vi "DemoApplication_Create.vi"(8 "Error In":errorcluster, 11 "reference in":refnum<class "DemoApplication.lvclass">) -> (0 "Error Out":errorcluster, 3 "reference out":refnum<class "DemoApplication.lvclass">)   [LabVIEW 2021, in "DemoApplication.lvclass"]
uses:
  DemoApplication.lvclass
  C:/Localdata/Projects/TriekselSoft/TriekselsoftApplicationFramework/Source/.Externals/Library_TAF_ApplicationFramework/MasterGUI/MasterGUI.lvclass
  .Externals/Library_TAF_ApplicationFramework/MasterGUI/MasterGUI.lvclass
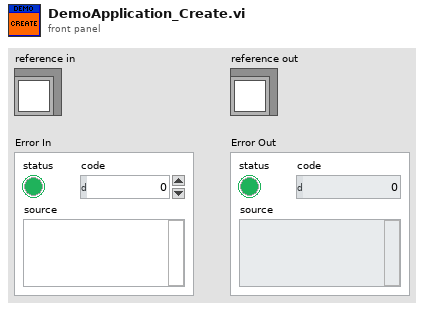
[diagram p1: front panel]
types:
  T1 = typedef "DemoApplication.lvclass/ObjectAttributes.ctl" = cluster{"Interfaces":cluster{"Authorizer":refnum<class "IAuthorization.lvclass">, "TextViewer":refnum<class "ITAFTextViewer.lvclass">, "ApplicationConfiguration":refnum<class "IApplicationConfiguration.lvclass">, "Tracer":refnum<class "IFrontPanel.lvclass">}, "Persistent":cluster{"MenuEnables":cluster{"MenuTag":string, "MenuExpression":string}[], "TextDockSubPanelName":string}}
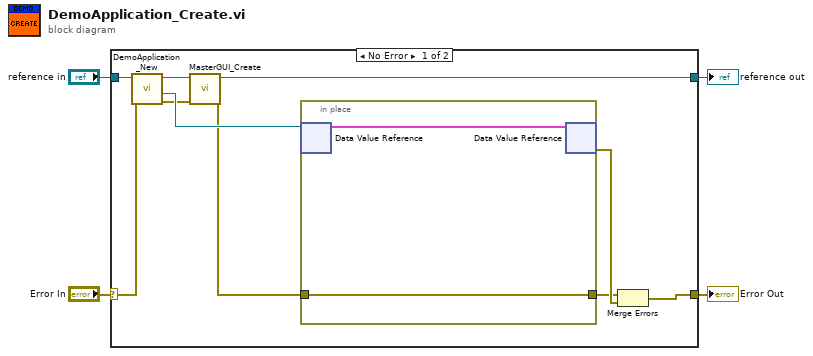
[diagram p0: block diagram]
diagram:
  n1 = case shown="No Error" "Error In" {
    selector: "Error In" -> [w13 w18]
    tunnel: [w8 w18] -> w3
    tunnel: "reference in" -> [w14 w17]
    tunnel: [w5 w17] -> w1
    frame No Error {
      n2 = call "DemoApplication_New.vi"("error in (no error)"=w13, "reference in"=w14) -> ("error out"=w10:errorcluster, "DVRRefOut"=w11:refnum<data-value>, "reference out"=w6:refnum<class "DemoApplication.lvclass">)  [unwired: 6 in, 1 out]
      n3 = call "MasterGUI_Create.vi"("Error In"=w10, "reference in"=w6) -> ("Error Out"=w7:errorcluster, "reference out"=w5:refnum<class "DemoApplication.lvclass">)  [unwired: 8 in]
      n4 = in-place {
        in-place-border: w7 -> [w16]
        in-place-border: [w16] -> w9
        n5 = in-place-dvr #1(w11) -> (w15:T1)  [unwired: 1 out]
        n6 = in-place-dvr #1(w15) -> (w12:errorcluster)  [unwired: 1 out]
      }
      n7 = Merge Errors(w9, w12) -> (w8:errorcluster)
    }
    frame Error {
      # "VI-TechBaseTemplate_Simple_4x4x4"
    }
  }
  "Error Out" <- w3
  "reference out" <- w1
